vi "Set Enable State on Multiple Controls(Cluster).vi"(8 "Enable?":bool, 11 "UI Refs":T1) -> (3 "UI Ref Out":T1)   [LabVIEW 2019]
doc: "Sets all the controls in the input array to the \"Enable state\" value."
uses:
  controls/UI Data.ctl
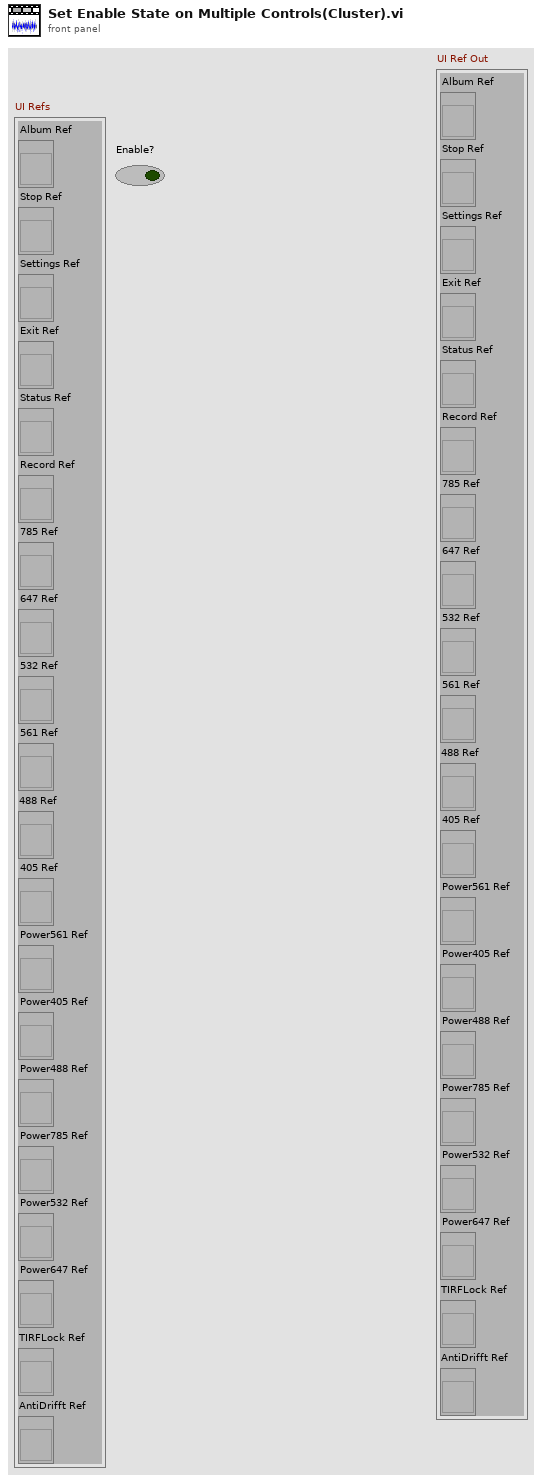
[diagram p1: front panel]
types:
  T1 = typedef "UI Data.ctl" = cluster{"Album Ref":refnum<vi>, "Stop Ref":refnum<vi>, "Settings Ref":refnum<vi>, "Exit Ref":refnum<vi>, "Status Ref":refnum<vi>, "Record Ref":refnum<vi>, "785 Ref":refnum<vi>, "647 Ref":refnum<vi>, "532 Ref":refnum<vi>, "561 Ref":refnum<vi>, "488 Ref":refnum<vi>, "405 Ref":refnum<vi>, "Power561 Ref":refnum<vi>, "Power405 Ref":refnum<vi>, "Power488 Ref":refnum<vi>, "Power785 Ref":refnum<vi>, "Power532 Ref":refnum<vi>, "Power647 Ref":refnum<vi>, "TIRFLock Ref":refnum<vi>, "AntiDrifft Ref":refnum<vi>}
  T2 = enum8{"Enabled", "Disabled", "Disabled and Grayed Out"}
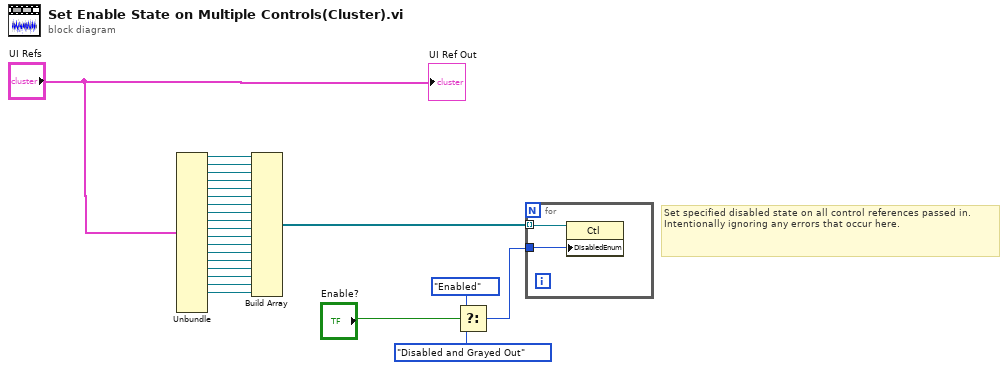
[diagram p0: block diagram]
diagram:
  # "Set specified disabled state on all control references passed in. Intentionally ignoring any errors that occur here."
  n1 = Unbundle("UI Refs") -> ("Album Ref"=w18:refnum<vi>, "Stop Ref"=w17:refnum<vi>, "Settings Ref"=w16:refnum<vi>, "Exit Ref"=w15:refnum<vi>, "Status Ref"=w14:refnum<vi>, "Record Ref"=w13:refnum<vi>, "785 Ref"=w12:refnum<vi>, "647 Ref"=w11:refnum<vi>, "532 Ref"=w10:refnum<vi>, "561 Ref"=w9:refnum<vi>, "488 Ref"=w8:refnum<vi>, "405 Ref"=w7:refnum<vi>, "Power561 Ref"=w6:refnum<vi>, "Power405 Ref"=w5:refnum<vi>, "Power488 Ref"=w4:refnum<vi>, "Power785 Ref"=w3:refnum<vi>, "Power532 Ref"=w2:refnum<vi>, "Power647 Ref"=w1:refnum<vi>)  [unwired: 2 out]
  n2 = Build Array(w18, w17, w16, w15, w14, w13, w12, w11, w10, w9, w8, w7, w6, w5, w4, w3, w2, w1) -> (w20:refnum<vi>[])
  n3 = Select(t=T2."Enabled" ("Disabled"), s="Enable?", f=T2."Disabled and Grayed Out" ("Disabled")) -> (s? t:f=w23:T2)
  n4 = for {
    tunnel: w20 -> [w26] mode=indexing
    tunnel: w23 -> [w25]
    n5 = property class="Ctl"(reference=w26, "DisabledEnum"=w25) -> ()  [unwired: 1 in, 2 out]
  }
  "UI Ref Out" <- "UI Refs"
